vi "Nick Config Tester.vi"() -> ()   [LabVIEW 2024]
uses:
  <vilib>/Utility/error.llb/Trim Whitespace One-Sided.vi
  <vilib>/Utility/config.llb/Read Key (String).vi
  <vilib>/Utility/config.llb/NI_LVConfig.lvlib
panel:
  out "match + rest of string 2":string
  out "substring before match 2":string
  out "substring before match":string
  out "match + rest of string":string
  out "text":string
  out "x = y?":bool
  out "Simulation value":string
  out "Simulation found?":bool
  out "error out":errorcluster
  out "Unitherm value":string
  out "Unitherm found?":bool
  in  "error in (no error)":errorcluster
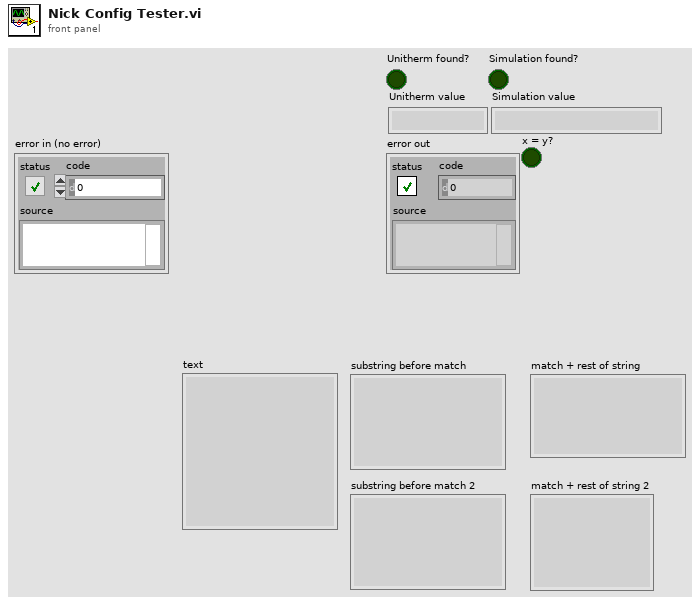
[diagram p1: front panel]
types:
  T1 = typedef "NI_LVConfig.lvlib/Config Data RefNum.ctl" = refnum<k1>
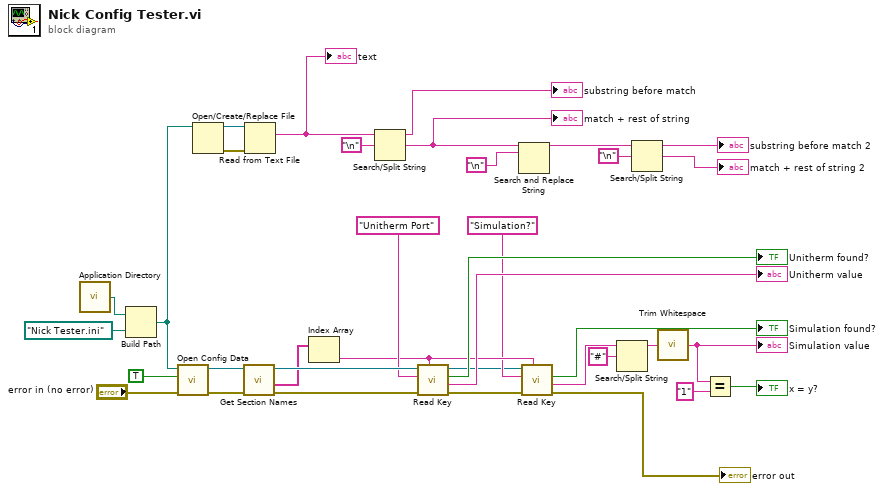
[diagram p0: block diagram]
diagram:
  n1 = call <vilib>:"Application Directory.vi"() -> ("Application Directory"=w32:path)
  n2 = Build Path(base path=w32, name or relative path=path "Nick Tester.ini") -> (appended path=w12:path)
  n3 = call <vilib>:"Open Config Data.vi"("error in (no error)"="error in (no error)", "create file if necessary (T)"=TRUE, "configuration file path"=w12) -> ("error out"=w33:errorcluster, "refnum"=w31:T1)  [unwired: 6 in, 1 out]
  n4 = Open/Create/Replace File(file path (use dialog)=w12) -> (refnum out=w10:refnum<file>, error out=w11:errorcluster)  [unwired: 5 in, 1 out]
  n5 = call <vilib>:"Get Section Names.vi"("error in (no error)"=w33, "refnum"=w31) -> ("error out"=w29:errorcluster, "section names"=w27:string[], "refnum out"=w30:T1)  [unwired: 7 in]
  n6 = Read from Text File(file (use dialog)=w10, error in=w11) -> (text=w9:string)  [unwired: 2 in, 3 out]
  "text" <- w9
  n7 = Index Array(array=w27) -> (element=w22:string)  [unwired: 1 in]
  n8 = Search/Split String(string=w9, search string/char (-)="\n") -> (substring before match=→"substring before match":string, match + rest of string=w5:string)  [unwired: 1 in, 1 out]
  "match + rest of string" <- w5
  n9 = call-poly <vilib>:"Read Key.vi"("section"=w22, "error in (no error)"=w29, "key"="Unitherm Port", "refnum"=w30) -> ("error out"=w24:errorcluster, "value"=→"Unitherm value":string, "found?"=→"Unitherm found?":bool, "refnum out"=w20:T1)  [unwired: 4 in]
  n10 = Search and Replace String(input string=w5, search string="\n") -> (result string=w2:string)  [unwired: 6 in, 3 out]
  n11 = call-poly <vilib>:"Read Key.vi"("section"=w22, "error in (no error)"=w24, "key"="Simulation?", "refnum"=w20) -> ("error out"=→"error out":errorcluster, "value"=w18:string, "found?"=→"Simulation found?":bool)  [unwired: 4 in, 1 out]
  n12 = Search/Split String(string=w18, search string/char (-)="#") -> (substring before match=w16:string)  [unwired: 1 in, 2 out]
  n13 = Search/Split String(string=w2, search string/char (-)="\n") -> (substring before match=→"substring before match 2":string, match + rest of string=→"match + rest of string 2":string)  [unwired: 1 in, 1 out]
  n14 = call <vilib>:"Trim Whitespace.vi"("string"=w16) -> ("trimmed string"=w13:string)  [unwired: 1 in]
  "Simulation value" <- w13
  n15 = Equal?(x=w13, y="1") -> (x = y?=→"x = y?":bool)
